vi "UDP发送.vi"(0 "发送数据":u16[](array[numeric]) format="%x", 1 "数据区字长":u16 format="%x", 2 "报文类型":u16 format="%x", 3 "发送方标识":u16 format="%x") -> (9 "Error":cluster{"错误？":bool, "数值":i32, "字符串":string})   [LabVIEW 2010]
uses:
  全局量/全局_配置.vi
panel:
  in  "校验码":u16 format="%x"
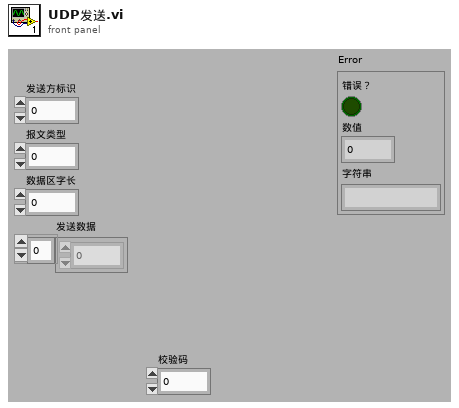
[diagram p1: front panel]
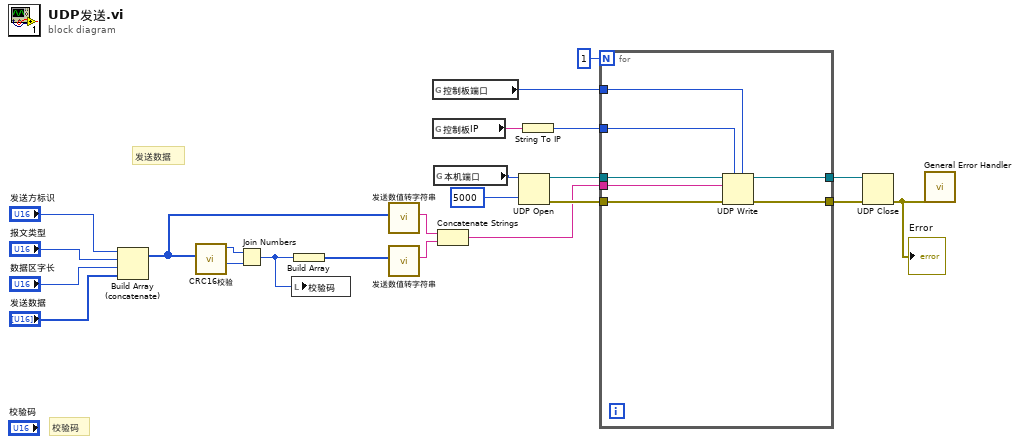
[diagram p0: block diagram]
diagram:
  # "校验码"
  # "发送数据"
  n1 = Build Array (concatenate)("发送方标识", "报文类型", "数据区字长", "发送数据") -> (w2:u16[])
  n2 = call "CRC16校验.vi"("输入数据_U16"=w2) -> ("低字节"=w22:u8, "高字节"=w23:u8)  [unwired: 9 in]
  n3 = Join Numbers(hi=w23, lo=w22) -> ((hi.lo)=w10:u16)
  n4 = local write "校验码"(w10) -> ()
  n5 = Build Array(w10) -> (w9:u16[])
  n6 = call "发送数值转字符串.vi"("输入数据_U16"=w2) -> ("字符串"=w12:string)  [unwired: 10 in]
  n7 = call "发送数值转字符串.vi"("输入数据_U16"=w9) -> ("字符串"=w11:string)  [unwired: 10 in]
  n8 = global read "全局_配置.vi" "控制板端口"() -> (w8:u16)
  n9 = global read "全局_配置.vi" "控制板IP"() -> (w6:string)
  n10 = global read "全局_配置.vi" "本机端口"() -> (w7:u16)
  n11 = Concatenate Strings(w12, w11) -> (w5:string)
  n12 = UDP Open(9:5000 ("超时毫秒(25000)"), 11:w7) -> (port=w17:refnum<k16>, 0:w18:errorcluster)  [unwired: 3 in, 1 out]
  n13 = String To IP(1:w6) -> (0:w21:u32)
  n14 = for {
    N: 1 -> [_]
    tunnel: w21 -> [w30]
    tunnel: [w29] -> w20
    tunnel: [w28] -> w19
    tunnel: w18 -> [w27]
    tunnel: w17 -> [w26]
    tunnel: w8 -> [w25]
    tunnel: w5 -> [w24]
    n15 = UDP Write(address=w30, port or service name=w25, connection ID=w26, data in=w24, 8:w27) -> (error out=w29:errorcluster, 3:w28:refnum<k16>)  [unwired: 1 in]
  }
  n16 = UDP Close(connection ID=w19, 8:w20) -> (error out=w4:errorcluster)  [unwired: 1 out]
  "Error" <- w4
  n17 = call <vilib>:"General Error Handler.vi"("error in (no error)"=w4) -> ()  [unwired: 10 in, 5 out]
